vi "NewErriorLoggerFile.vi"(8 "error in (no error)":errorcluster, 9 "ErrorLogPath":path, 10 "Filenumber":u32, 11 "TCP_Server in":refnum<class "TCP_Server.lvclass">) -> (0 "error out":errorcluster, 3 "TCP_Server out":refnum<class "TCP_Server.lvclass">)   [LabVIEW 2023, in "TCP_Server.lvlib" / "TCP_Server.lvclass"]
uses:
  TCP_Server.lvclass
  TCP_Server.lvclass/TCP_Server.ctl
  TCP_serverGUI/TCP_serverGUI Messages/UpdateErrorfile Msg/UpdateErrorfile Msg.lvclass
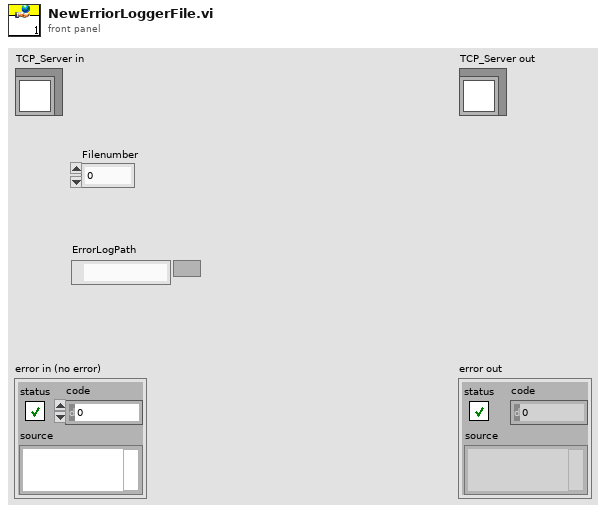
[diagram p1: front panel]
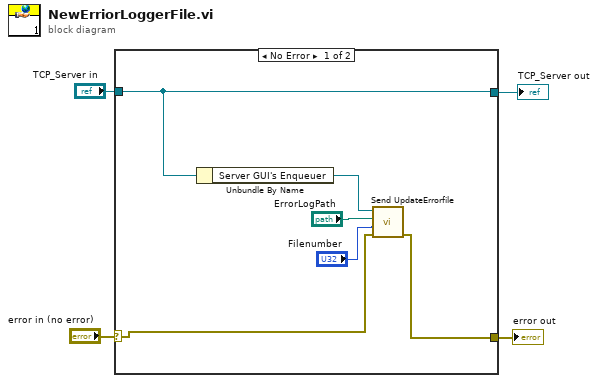
[diagram p0: block diagram]
diagram:
  n1 = case shown="No Error" "error in (no error)" {
    selector: "error in (no error)" -> [w7 w12]
    tunnel: [w6 w12] -> w3
    tunnel: "TCP_Server in" -> [w5 w11]
    tunnel: [w5 w11] -> w1
    frame No Error {
      n2 = Unbundle By Name(w5) -> ("Server GUI's Enqueuer"=w10:refnum<class "Message Enqueuer.lvclass">)
      n3 = call "Send UpdateErrorfile.vi"("error in (no error)"=w7, "Error file number"="Filenumber", "Error file"="ErrorLogPath", "Message Enqueuer"=w10) -> ("error out"=w6:errorcluster)  [unwired: 6 in, 1 out]
    }
    frame Error {
    }
  }
  "error out" <- w3
  "TCP_Server out" <- w1
